vi "rotate_about_principal_axis.vi"(7 "axis":T1, 8 "error in (no error)":errorcluster, 10 "angle":dbl[unit], 11 "PointCollection in":refnum<class "PointCollection.lvclass">) -> (0 "error out":errorcluster, 3 "PointCollection out":refnum<class "PointCollection.lvclass">)   [LabVIEW 2010, in "PointCollection.lvclass"]
uses:
  PointCollection.lvclass
  x_y_z_enumeration.ctl
  PointCollection.lvclass/PointCollection.ctl
  mode_enum.ctl
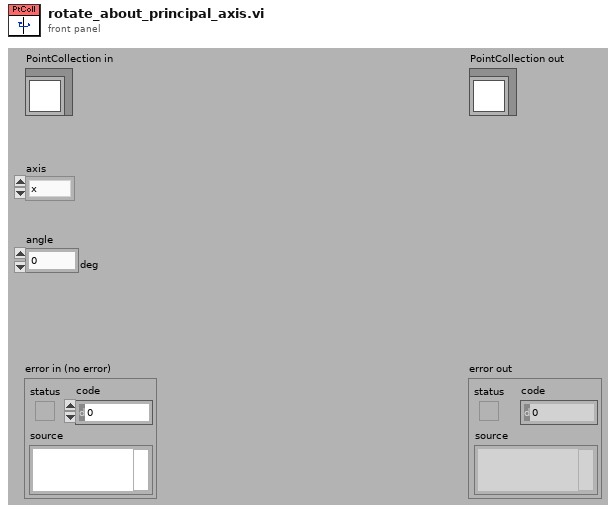
[diagram p1: front panel]
types:
  T1 = typedef "PointCollection.lvclass/x_y_z_enumeration.ctl" = enum16{"x", "y", "z"}
  T2 = typedef "PointCollection.lvclass/mode_enum.ctl" = enum16{"points first", "dimensions first"}
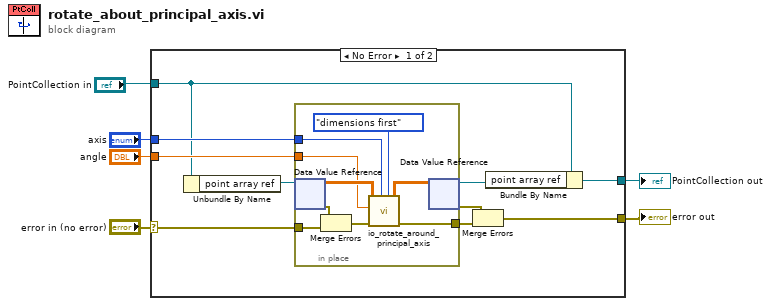
[diagram p0: block diagram]
diagram:
  n1 = case shown="No Error" "error in (no error)" {
    selector: "error in (no error)" -> [w16 w27]
    tunnel: [w9 w27] -> w5
    tunnel: [w8 w26] -> w1
    tunnel: "angle" -> [w13 _]
    tunnel: "axis" -> [w14 _]
    tunnel: "PointCollection in" -> [w10 w26]
    frame No Error {
      n2 = Unbundle By Name(w10) -> ("point array ref"=w15:refnum<data-value>)
      n3 = in-place {
        in-place-border: w16 -> [w23]
        in-place-border: w14 -> [w21]
        in-place-border: w13 -> [w20]
        in-place-border: [w18] -> w11
        n4 = in-place-dvr #1(w15) -> (w25:dbl[][], w24:errorcluster)
        n5 = Merge Errors(w24, w23) -> (w22:errorcluster)
        n6 = call "io_rotate_around_principal_axis.vi"("mode"=mode_enum."dimensions first", "axis"=w21, "error in (no error)"=w22, "angle"=w20, "points in"=w25) -> ("error out"=w18:errorcluster, "points out"=w19:dbl[][])  [unwired: 5 in]
        n7 = in-place-dvr #1(w19) -> (w7:refnum<data-value>, w12:errorcluster)
      }
      n8 = Merge Errors(w12, w11) -> (w9:errorcluster)
      n9 = Bundle By Name(cluster=w10, "point array ref"=w7) -> (w8:refnum<class "PointCollection.lvclass">)
    }
    frame Error {
    }
  }
  "error out" <- w5
  "PointCollection out" <- w1
